vi "WLAN_be_EVM_SG.vi"(5 "Function_SG":T1, 7 "setPower":i32, 8 "error in":errorcluster, 11 "VISA IN":refnum<visa-resource-name>="IQGIG") -> (0 "error out":errorcluster, 3 "IDN":string)   [LabVIEW 2023, in "LitePoints.lvlib"]
uses:
  LitePoints.lvlib
  CTL/LitePoint_EVM_SG.ctl
panel:
  out "Response":string
  # "IQgig-5G : TCPIP0::192.168.100.254::hislip0::INSTR"
  # "IQxel-MX : TCPIP0::192.168.100.253::hislip0::INSTR"
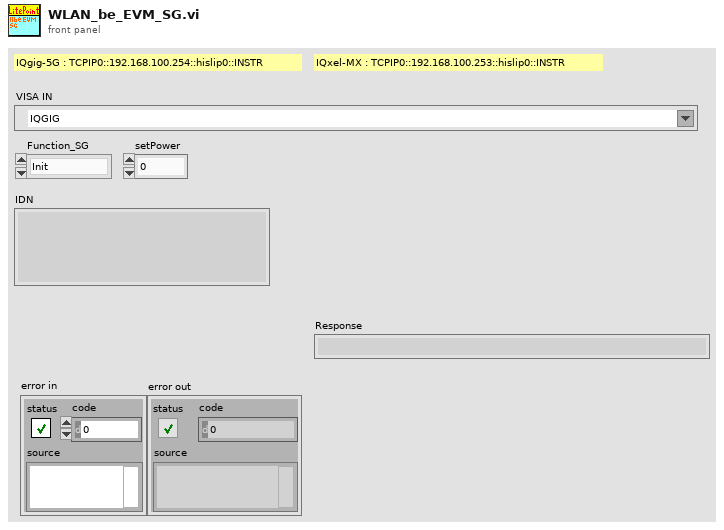
[diagram p1: front panel]
types:
  T1 = typedef "LitePoint_EVM_SG.ctl" = enum16{"Init", "Close", "set_SG", "AdjustLevel", "byPass", "RF_ON", "RF_OFF"}
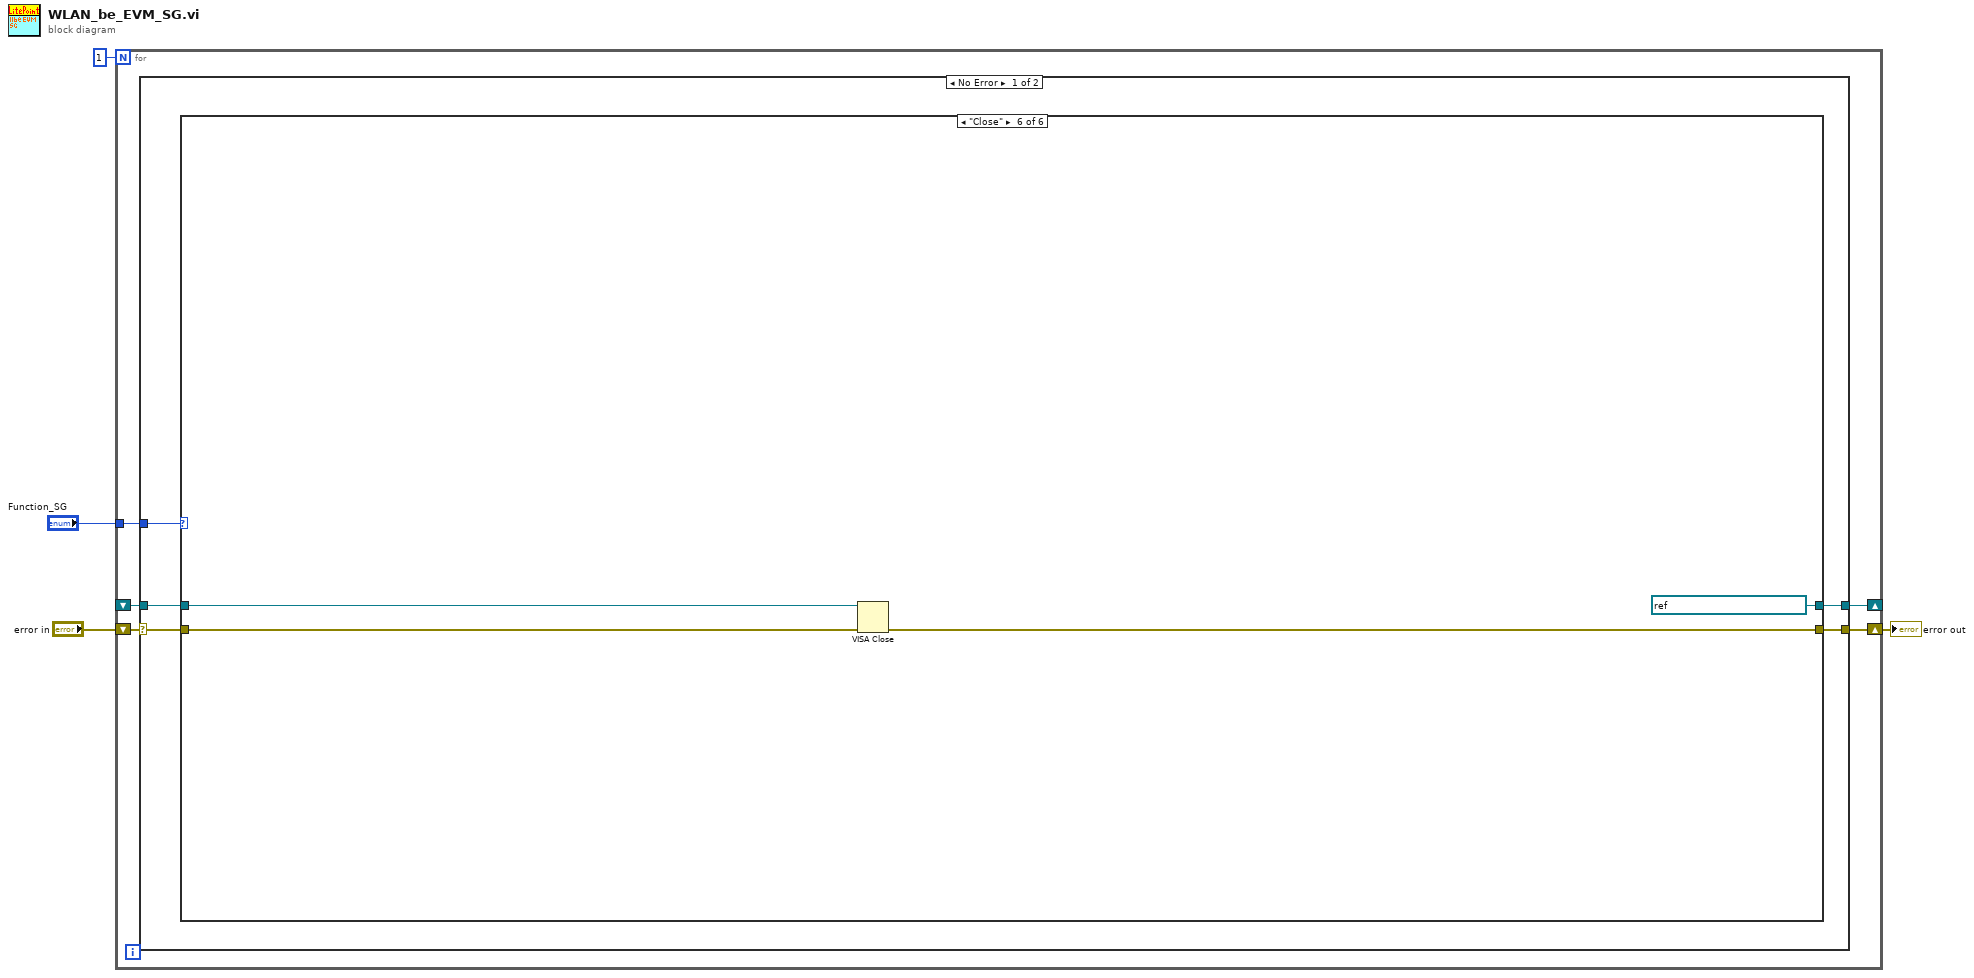
[diagram p0: block diagram]
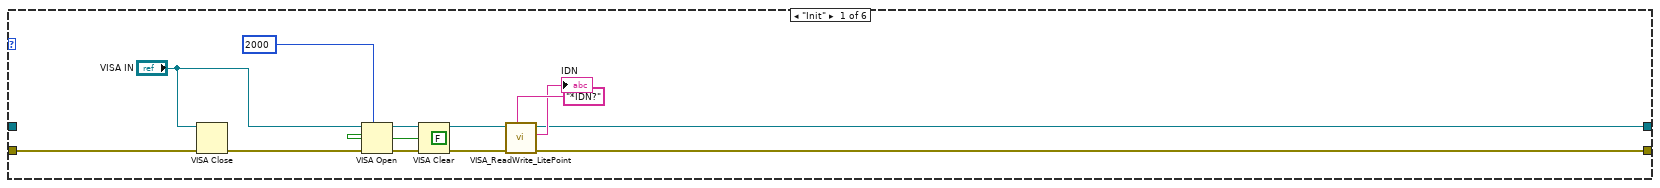
[diagram p2: hidden frame]
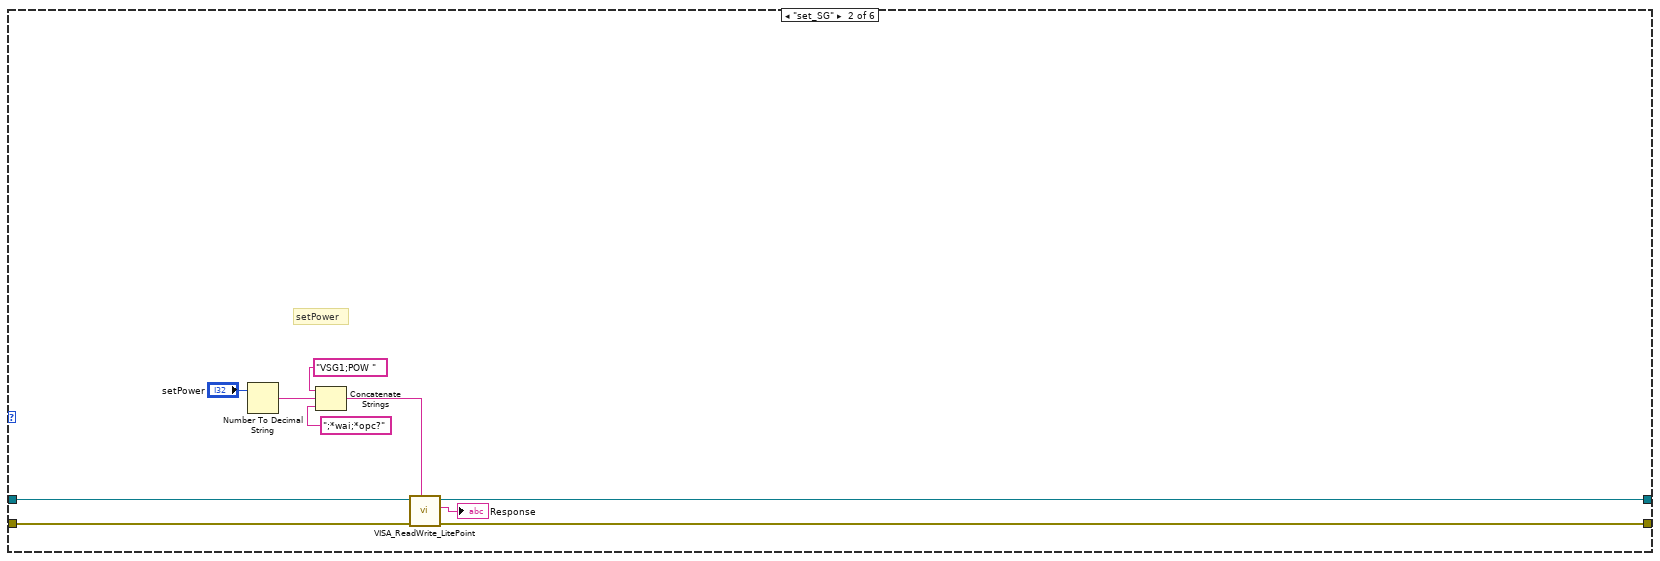
[diagram p3: hidden frame]
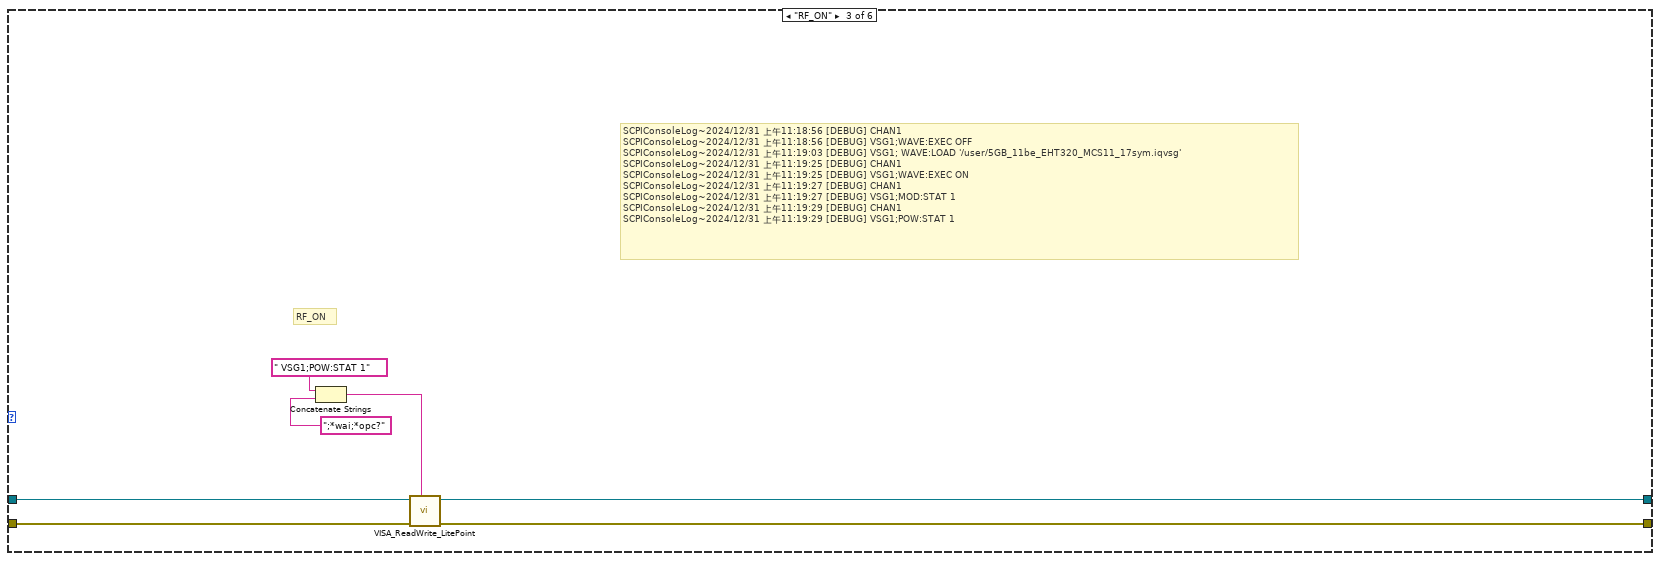
[diagram p4: hidden frame]
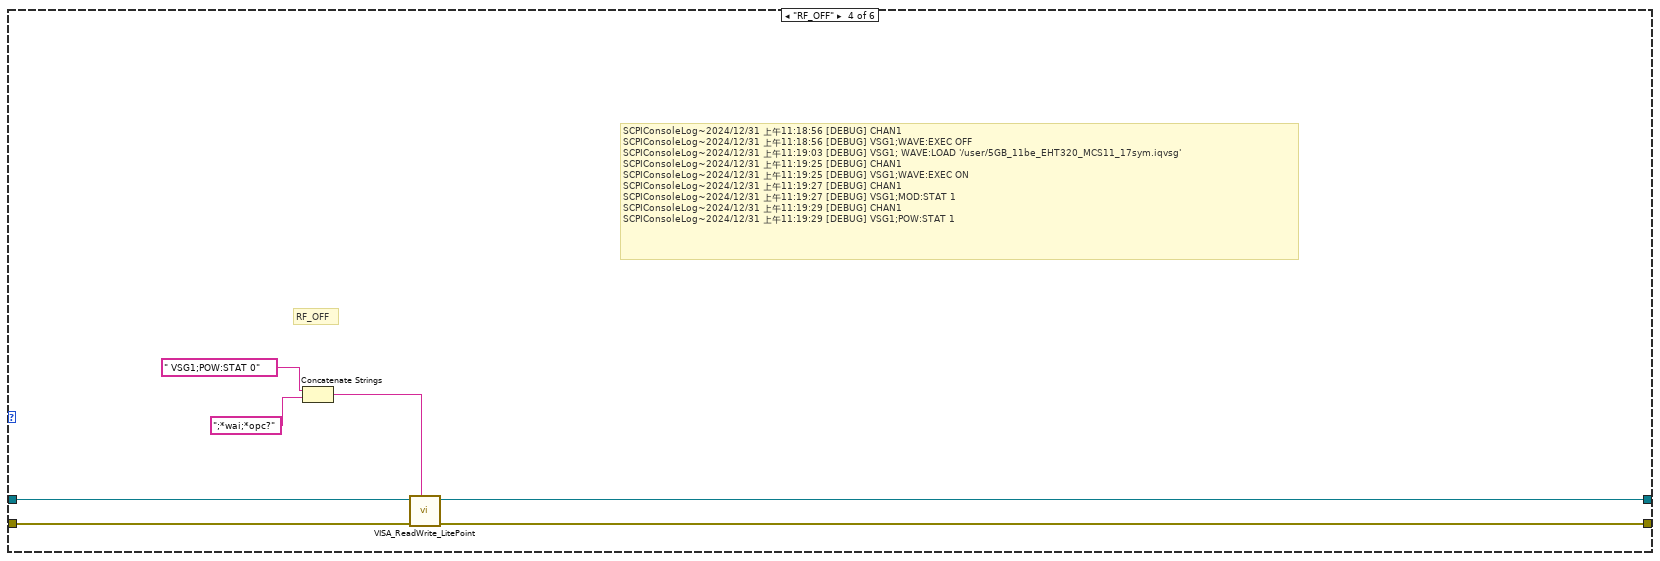
[diagram p5: hidden frame]
diagram:
  n1 = for {
    N: 1 -> [_]
    tunnel: "Function_SG" -> [w7]
    shift-right: [w8] -> w3
    shift-left: "error in" -> [w9]
    shift-right: [w5] -> _
    shift-left: _ -> [w6]
    n2 = case shown="No Error" w9 {
      selector: w9 -> [w13 w59]
      tunnel: [w12 w59] -> w8
      tunnel: w7 -> [w14 _]
      tunnel: w6 -> [w11 w58]
      tunnel: [w10 w58] -> w5
      frame No Error {
        n3 = case shown="\"Close\"" w14 {
          tunnel: [w22 w28 w39 w48 w53 w57] -> w12
          tunnel: w13 -> [w17 w32 w42 w50 w53 w56]
          tunnel: w11 -> [_ w33 w43 w51 w52 w55]
          tunnel: [w18 w29 w40 w49 w52 refnum<visa-resource-name> refnum ("VISA out")] -> w10
          frame "Init" {
            n4 = VISA Close(VISA resource name="VISA IN", error in (no error)=w17) -> (error out=w16:errorcluster)
            n5 = VISA Open(timeout (0)=u32 2000 ("VISA Open timeout (0)"), duplicate session (F)=FALSE, error in (no error)=w16, VISA resource name="VISA IN") -> (VISA resource name=w24:refnum<visa-resource-name>, error out=w25:errorcluster)  [unwired: 1 in]
            n6 = VISA Clear(VISA resource name=w24, error in (no error)=w25) -> (VISA resource name out=w21:refnum<visa-resource-name>, error out=w23:errorcluster)
            n7 = call "VISA_ReadWrite_LitePoint.vi"("VISA_CMD"="*IDN?", "error in"=w23, "VISA in"=w21) -> ("error out"=w22:errorcluster, "Response"=→"IDN":string, "VISA out"=w18:refnum<visa-resource-name>)  [unwired: 6 in]
          }
          frame "set_SG" {
            # "setPower"
            n8 = Number To Decimal String(number="setPower") -> (decimal integer string=w37:string)  [unwired: 1 in]
            n9 = Concatenate Strings("VSG1;POW " ("write buffer"), w37, ";*wai;*opc?" ("write buffer")) -> (w31:string)
            n10 = call "VISA_ReadWrite_LitePoint.vi"("VISA_CMD"=w31, "error in"=w32, "VISA in"=w33) -> ("error out"=w28:errorcluster, "Response"=→"Response":string, "VISA out"=w29:refnum<visa-resource-name>)  [unwired: 6 in]
          }
          frame "RF_ON" {
            # "SCPIConsoleLog~2024/12/31 上午11:18:56 [DEBUG] CHAN1\nSCPIConsoleLog~2024/12/31 上午11:18:56 [DEBUG] VSG1;WAVE:EXEC OFF\nSCPIConsoleLog~2024/12/31 上午11:19:03 [DEBUG] VSG1; WAVE:LOAD '/user/5GB_11be_EHT320_MCS11_17sym.iqvsg'\nSCPIConsoleLog~2024/12/31 上午11:19:25 [DEBUG] CHAN1\nSCPIConsoleLog~2024/12/31 上午11:19:25 [DEBUG] VSG1;WAVE:EXEC ON\nSCPIConsoleLog~2024/12/31 上午11:19:27 [DEBUG] CHAN1\nSCPIConsoleLog~2024/12/31 上午11:19:27 [DEBUG] VSG1;MOD:STAT 1\nSCPIConsoleLog~2024/12/31 上午11:19:29 [DEBUG] CHAN1\nSCPIConsoleLog~2024/12/31 上午11:19:29 [DEBUG] VSG1;POW:STAT 1"
            # "RF_ON"
            n11 = Concatenate Strings(" VSG1;POW:STAT 1" ("write buffer"), ";*wai;*opc?" ("write buffer")) -> (w41:string)
            n12 = call "VISA_ReadWrite_LitePoint.vi"("VISA_CMD"=w41, "error in"=w42, "VISA in"=w43) -> ("error out"=w39:errorcluster, "VISA out"=w40:refnum<visa-resource-name>)  [unwired: 6 in, 1 out]
          }
          frame "RF_OFF" {
            # "SCPIConsoleLog~2024/12/31 上午11:18:56 [DEBUG] CHAN1\nSCPIConsoleLog~2024/12/31 上午11:18:56 [DEBUG] VSG1;WAVE:EXEC OFF\nSCPIConsoleLog~2024/12/31 上午11:19:03 [DEBUG] VSG1; WAVE:LOAD '/user/5GB_11be_EHT320_MCS11_17sym.iqvsg'\nSCPIConsoleLog~2024/12/31 上午11:19:25 [DEBUG] CHAN1\nSCPIConsoleLog~2024/12/31 上午11:19:25 [DEBUG] VSG1;WAVE:EXEC ON\nSCPIConsoleLog~2024/12/31 上午11:19:27 [DEBUG] CHAN1\nSCPIConsoleLog~2024/12/31 上午11:19:27 [DEBUG] VSG1;MOD:STAT 1\nSCPIConsoleLog~2024/12/31 上午11:19:29 [DEBUG] CHAN1\nSCPIConsoleLog~2024/12/31 上午11:19:29 [DEBUG] VSG1;POW:STAT 1"
            # "RF_OFF"
            n13 = Concatenate Strings(" VSG1;POW:STAT 0" ("write buffer"), ";*wai;*opc?" ("write buffer")) -> (w47:string)
            n14 = call "VISA_ReadWrite_LitePoint.vi"("VISA_CMD"=w47, "error in"=w50, "VISA in"=w51) -> ("error out"=w48:errorcluster, "VISA out"=w49:refnum<visa-resource-name>)  [unwired: 6 in, 1 out]
          }
          frame "byPass", Default {
          }
          frame "Close" {
            n15 = VISA Close(VISA resource name=w55, error in (no error)=w56) -> (error out=w57:errorcluster)
          }
        }
      }
      frame Error {
      }
    }
  }
  "error out" <- w3
